vi "RC_Client Client.vi"(8 "error in (no error)":errorcluster, 11 "RemoteControl in":refnum<class "RemoteControl.lvclass">) -> (0 "error out":errorcluster)   [LabVIEW 2019, in "RemoteControl.lvclass"]
uses:
  RemoteControl.lvclass
  9c1bb9c7-6493-4123-b83c-24e0bfa81f7e.vi
panel:
  in  "milliseconds to wait":u32
  out "time (1 message) (ms)":u32
  out "messsages/s":dbl
  in  "remote port":u16=6341
  in  "address":string
  out "Parse Response":string
  out "Messages":i32
  in  "Stop":bool
  out "Command reponse":string
  out "Command":string
  out "commands":string[](array[string])
  # "CLIENT (API)"
  # "Connection info"
  # "Message Sent"
  # "Message Received"
  # "Metrics"
  # "client 1"
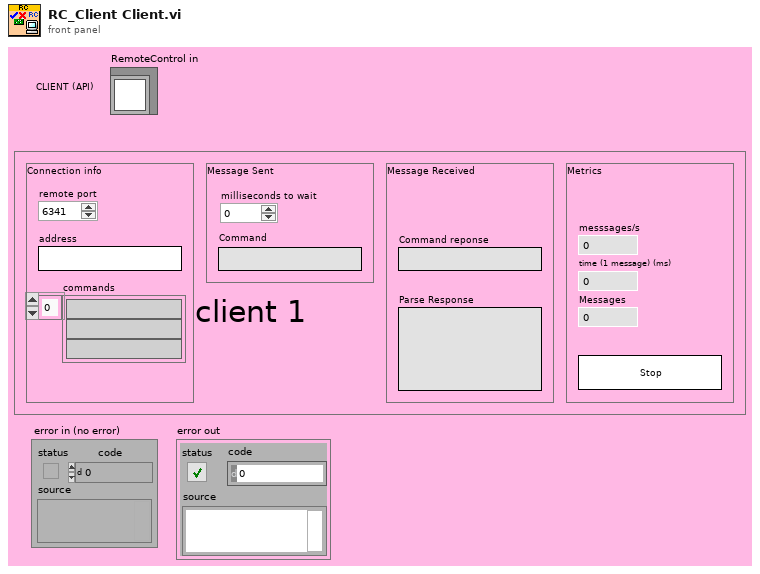
[diagram p1: front panel]
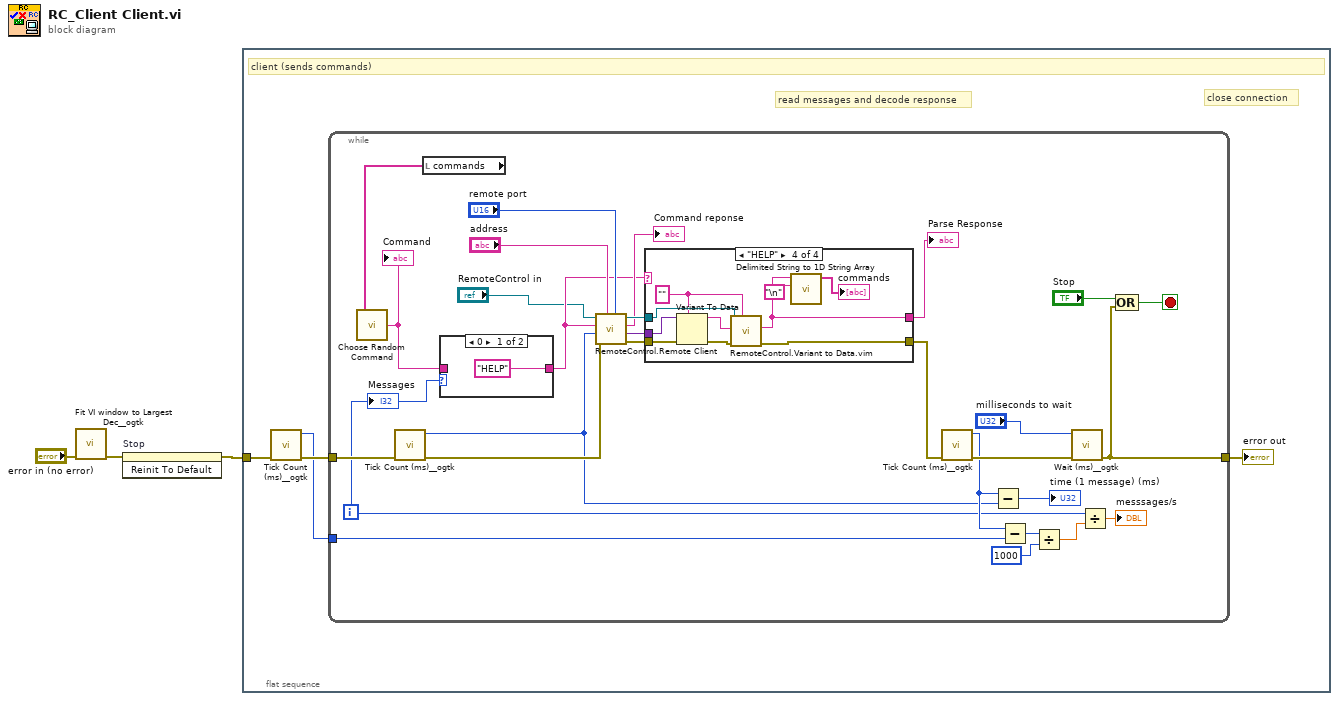
[diagram p0: block diagram]
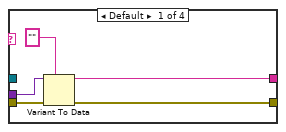
[diagram p3: hidden frame]
diagram:
  n1 = call <userlib>:"Fit VI window to Largest Dec__ogtk.vi"("error in (no error)"="error in (no error)") -> ("error out"=w3:errorcluster)  [unwired: 5 in, 1 out]
  n2 = invoke on="Stop" class="Bool" method="Reinit To Default"(error in=w3) -> (error out=w2:errorcluster)  [unwired: 2 in, 2 out]
  n3 = flat-sequence {
    tunnel: w2 -> [w4]
    frame #0 {
      # "close connection"
      # "read messages and decode response"
      # "client (sends commands)"
      n4 = call <userlib>:"Tick Count (ms)__ogtk.vi"("error in (no error)"=w4) -> ("error out"=w7:errorcluster, "millisecond timer value"=w6:u32)  [unwired: 9 in]
      n5 = while {
        tunnel: [w29] -> w5
        tunnel: w7 -> [w32]
        tunnel: w6 -> [w24]
        i -> [w16]
        stop <- w35 stop-if-true
        n6 = call <userlib>:"Tick Count (ms)__ogtk.vi"("error in (no error)"=w32) -> ("error out"=w20:errorcluster, "millisecond timer value"=w9:u32)  [unwired: 9 in]
        n7 = local read "commands"() -> (w13:string[])
        n8 = call "Choose Random Command.vi"("Array"=w13) -> ("String"=w12:string)
        "Command" <- w12
        n9 = case shown="0" w16 {
          tunnel: ["HELP" ("Command") w37] -> w10
          tunnel: w12 -> [_ w37]
          frame 0 {
          }
          frame Default {
          }
        }
        n10 = call "RemoteControl.Remote Client.vi"("Port"="remote port", "address"="address", "error in (no error)"=w20, "Data"=w9, "Command"=w10, "RemoteControl in"="RemoteControl in") -> ("error out"=w19:errorcluster, "Data out"=w21:variant, "Command out"=→"Command reponse":string, "RemoteControl out"=w23:refnum<class "RemoteControl.lvclass">)  [unwired: 2 in]
        n11 = case shown="\"HELP\"" w10 {
          selector: w10 -> [_ w43 w45 _]
          tunnel: [w38 w43 w45 w47] -> w18
          tunnel: w23 -> [_ _ _ w50]
          tunnel: w21 -> [w42 _ _ w56]
          tunnel: [w39 w44 w46 w48] -> w17
          tunnel: w19 -> [w40 w44 w46 w55]
          frame Default {
            n12 = Variant To Data(error in=w40, type="", Variant=w42) -> (data=w38:string, error out=w39:errorcluster)
          }
          frame "open" {
          }
          frame "close" {
          }
          frame "HELP" {
            w49 = ""
            n13 = Variant To Data(error in=w55, type=w49, Variant=w56) -> (data=w51:string, error out=w52:errorcluster)
            n14 = call "RemoteControl.Variant to Data.vim"("Data Type"=w49, "error in (no error)"=w52, "Data in"=w51, "RemoteControl in"=w50) -> ("error out"=w48:errorcluster, "Data out"=w47:string)  [unwired: 5 in, 1 out]
            n15 = call <vilib>:"Delimited String to 1D String Array.vi"("delimiter"="\n", "delimited string"=w47) -> ("string array"=→"commands":string[])  [unwired: 9 in]
          }
        }
        "Parse Response" <- w18
        n16 = call <userlib>:"Tick Count (ms)__ogtk.vi"("error in (no error)"=w17) -> ("error out"=w31:errorcluster, "millisecond timer value"=w26:u32)  [unwired: 9 in]
        n17 = Subtract(x=w26, y=w9) -> (x-y=→"time (1 message) (ms)":u32)
        n18 = Subtract(x=w26, y=w24) -> (x-y=w25:u32)
        n19 = Divide(x=w25, y=u32 1000) -> (x/y=w34:dbl)
        n20 = call <userlib>:"Wait (ms)__ogtk.vi"("error in (no error)"=w31, "milliseconds to wait"="milliseconds to wait") -> ("error out"=w29:errorcluster)  [unwired: 8 in, 1 out]
        n21 = Divide(x=w16, y=w34) -> (x/y=→"messsages/s":dbl)
        n22 = Compound Arithmetic op=OR("Stop", w29) -> (w35:bool)
        "Messages" <- w16
      }
      "error out" <- w5
    }
  }
